vi "Inst.Krohn-Hite-7008.DoSomething.vi"(8 "error in (no error)":errorcluster, 10 "Data":variant, 11 "Inst.Krohn-Hite-7008 in":refnum<class "Inst.Krohn-Hite-7008.lvclass">) -> (0 "error out":errorcluster, 2 "Data out":variant, 3 "Inst.Krohn-Hite-7008 out":refnum<class "Inst.Krohn-Hite-7008.lvclass">)   [LabVIEW 2019, in "Inst.Krohn-Hite-7008.lvclass"]
uses:
  Inst.Krohn-Hite-7008.lvclass
  Inst.Krohn-Hite-7008.lvclass/Inst.Krohn-Hite-7008.ctl
  fdab1b40-c942-4d42-9f74-5965e28da6e4.vi
  <vilib>/JDP Science/JSONtext/JSON text to Variant.vi
  <vilib>/JDP Science/JSONtext/LVClass Serializer/JSONtext LVClass Serializer.lvclass
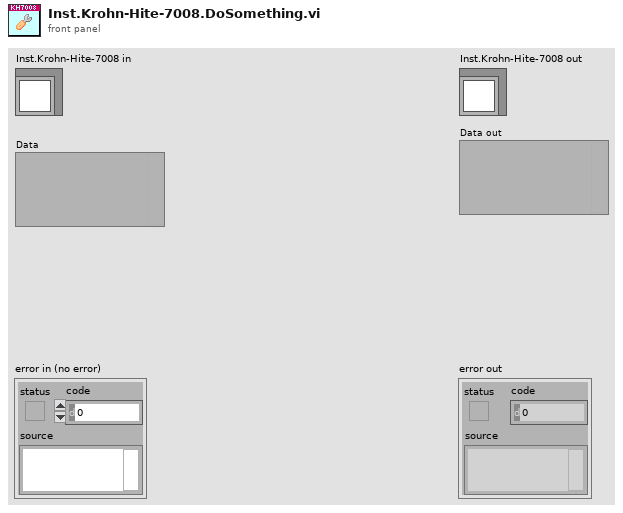
[diagram p1: front panel]
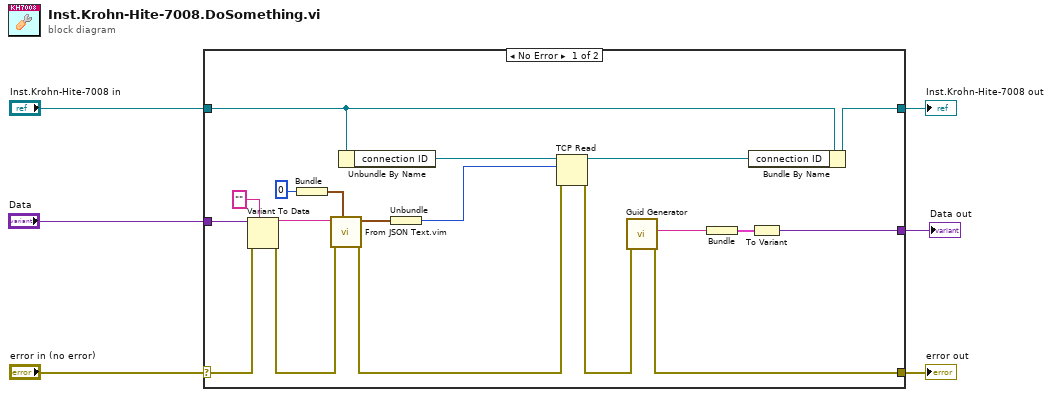
[diagram p0: block diagram]
diagram:
  n1 = case shown="No Error" "error in (no error)" {
    selector: "error in (no error)" -> [w19 w27]
    tunnel: [w9 w27] -> w5
    tunnel: [w25 w26] -> w3
    tunnel: "Inst.Krohn-Hite-7008 in" -> [w24 w26]
    tunnel: "Data" -> [w21 _]
    tunnel: [w8 _] -> w1
    frame No Error {
      n2 = Variant To Data(error in=w19, type="", Variant=w21) -> (data=w18:string, error out=w17:errorcluster)
      n3 = Bundle("bytes to read"=0) -> (w15:cluster{"bytes to read":i32})  [unwired: 1 in]
      n4 = call "From JSON Text.vim"("Data Type and Default Value"=w15, "error in (no error)"=w17, "JSON"=w18) -> ("error out"=w16:errorcluster, "Data out"=w14:cluster{"bytes to read":i32})  [unwired: 7 in]
      n5 = Unbundle By Name(w24) -> ("connection ID"=w23:refnum<k5>)
      n6 = Unbundle(w14) -> ("bytes to read"=w13:i32)
      n7 = TCP Read(connection ID=w23, bytes to read=w13, error in (no error)=w16) -> (connection ID out=w22:refnum<k5>, error out=w10:errorcluster)  [unwired: 2 in, 1 out]
      n8 = call <vilib>:"Guid Generator.vi"("error in (no error)"=w10) -> ("error out"=w9:errorcluster, "GUID"=w11:string)  [unwired: 9 in]
      n9 = Bundle("GUID"=w11) -> (w7:cluster{"GUID":string})  [unwired: 1 in]
      n10 = Bundle By Name(cluster=w24, "connection ID"=w22) -> (w25:refnum<class "Inst.Krohn-Hite-7008.lvclass">)
      n11 = To Variant(anything=w7) -> (Variant=w8:variant)
    }
    frame Error {
    }
  }
  "error out" <- w5
  "Inst.Krohn-Hite-7008 out" <- w3
  "Data out" <- w1
